vi "Stop Heat.vi"(8 "error in (no error)":errorcluster, 11 "Ramp Oven in":refnum<class "Ramp Oven.lvclass">) -> (0 "error out":errorcluster, 3 "Ramp Oven out":refnum<class "Ramp Oven.lvclass">)   [LabVIEW 2021, in "Oven Actor.lvlib" / "Ramp Oven.lvclass"]
uses:
  Ramp Oven.lvclass
  <vilib>/ActorFramework/Actor/Actor.lvclass
  Cooker Actor/Cooker Actor Messages/Update Cooker Fire Msg/Update Cooker Fire Msg.lvclass
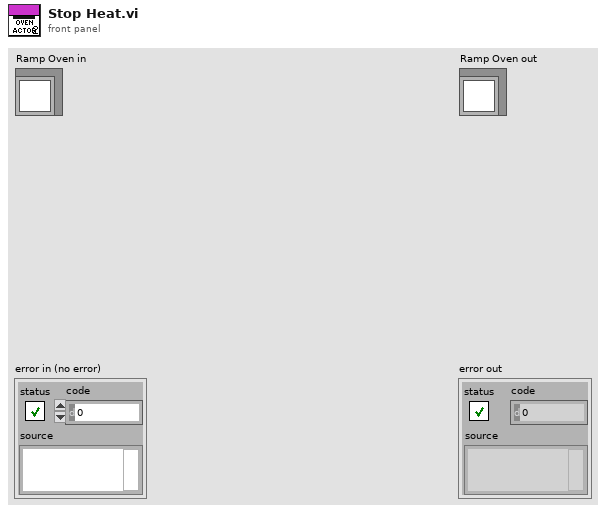
[diagram p1: front panel]
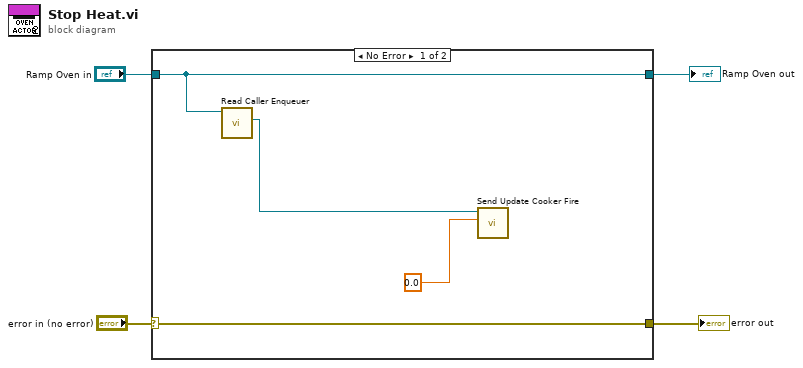
[diagram p0: block diagram]
diagram:
  n1 = case shown="No Error" "error in (no error)" {
    selector: "error in (no error)" -> [w6 w9]
    tunnel: [w6 w9] -> w3
    tunnel: "Ramp Oven in" -> [w5 w10]
    tunnel: [w5 w10] -> w1
    frame No Error {
      n2 = call <vilib>:"Read Caller Enqueuer.vi"("Actor"=w5) -> ("Caller Enqueuer"=w8:refnum<class "Message Enqueuer.lvclass">)  [unwired: 10 in]
      n3 = call "Send Update Cooker Fire.vi"("Fire (%)"=0.0, "Message Enqueuer"=w8) -> ()  [unwired: 8 in, 2 out]
    }
    frame Error {
    }
  }
  "error out" <- w3
  "Ramp Oven out" <- w1
